vi "array_generator.vi"(0 "Temp control parameters":T1 {"End Temp" format="%.2f"; "Temp Step" format="%.2f"; "Start Temp" format="%.2f"}) -> (1 "Temp array":dbl[](array[numeric]), 2 "N temps":dbl, 3 "Temp control parameters out":T1 {"End Temp" format="%.2f"; "Temp Step" format="%.2f"; "Start Temp" format="%.2f"})   [LabVIEW 2016]
doc: "This vi creates an array using the tempereture control parameters.\n\nInputs:\nTemp control parameters.\n\nOutputs:\nN temps,\nTemp array,\nTemp control parameters out.\n\nMuhannad Alghamdi\nCSUSB Physics 350"
uses:
  typedefs/temp_control_params.ctl
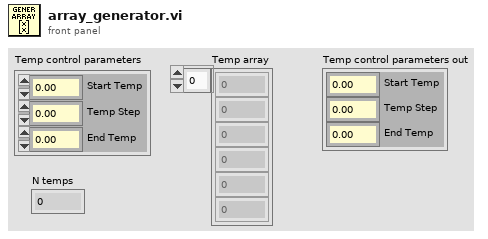
[diagram p1: front panel]
types:
  T1 = typedef "temp_control_params.ctl" = cluster{"Start Temp":dbl, "Temp Step":dbl, "End Temp":dbl}
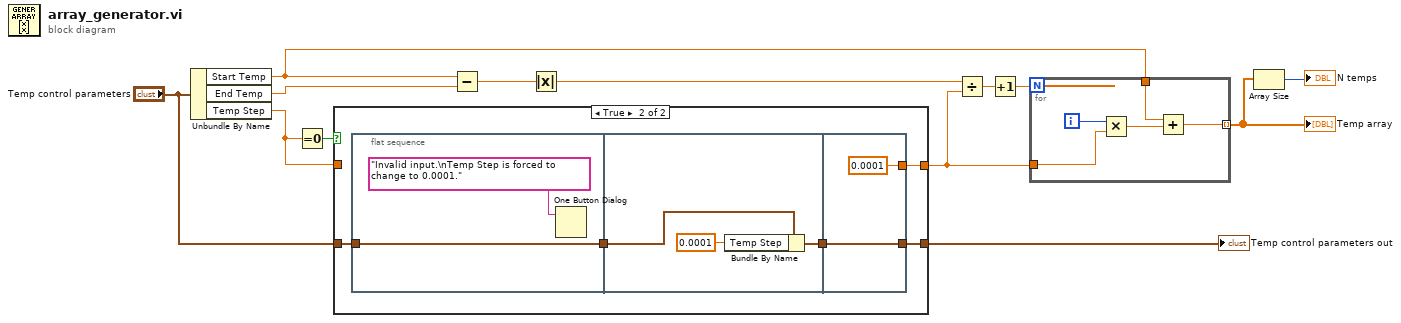
[diagram p0: block diagram]
diagram:
  n1 = Unbundle By Name("Temp control parameters") -> ("Start Temp"=w9:dbl, "End Temp"=w11:dbl, "Temp Step"=w6:dbl)
  n2 = Equal To 0?(x=w6) -> (x = 0?=w7:bool)
  n3 = case shown="True" w7 {
    tunnel: w6 -> [w15 _]
    tunnel: [w15 w20] -> w5
    tunnel: [w14 w18] -> w2
    tunnel: "Temp control parameters" -> [w14 w16]
    frame False {
    }
    frame True {
      n4 = flat-sequence {
        tunnel: [w21] -> w17
        tunnel: w16 -> [w21]
        tunnel: [w24] -> w19
        tunnel: w17 -> [w23]
        tunnel: [0.0001] -> w20
        tunnel: w19 -> [w26]
        tunnel: [w26] -> w18
        frame #0 {
          n5 = One Button Dialog(message="Invalid input.\nTemp Step is forced to change to 0.0001.") -> ()  [unwired: 1 in, 1 out]
        }
        frame #1 {
          n6 = Bundle By Name(cluster=w23, "Temp Step"=0.0001) -> (w24:T1)
        }
        frame #2 {
        }
      }
    }
  }
  "Temp control parameters out" <- w2
  n7 = Subtract(x=w9, y=w11) -> (x-y=w13:dbl)
  n8 = Absolute Value(x=w13) -> (abs(x)=w12:dbl)
  n9 = Divide(x=w12, y=w5) -> (x/y=w10:dbl)
  n10 = Increment(x=w10) -> (x+1=w8:dbl)
  n11 = for {
    N: w8 -> [_]
    tunnel: w9 -> [w30]
    tunnel: [w29] -> w3 mode=indexing
    tunnel: w5 -> [w28]
    i -> [w32]
    n12 = Multiply(x=w32, y=w28) -> (x*y=w31:dbl)
    n13 = Add(x=w30, y=w31) -> (x+y=w29:dbl)
  }
  "Temp array" <- w3
  n14 = Array Size(array=w3) -> (size(s)=→"N temps":i32)
